vi "Get Sub Objects.vi"(8 "error in":errorcluster, 11 "Sub Objects Dictionary in":refnum<class "Sub Objects Dictionary.lvclass">) -> (0 "error out":errorcluster, 2 "Sub Objects":refnum<class "Sub Object.lvclass">[](array[class]), 3 "Sub Objects Dictionary out":refnum<class "Sub Objects Dictionary.lvclass">)   [LabVIEW 2020, in "CANopen.lvlib" / "Sub Objects Dictionary.lvclass"]
uses:
  Sub Objects Dictionary.lvclass
  Sub Objects Dictionary.lvclass/Sub Objects Dictionary.ctl
  Sub Object/Sub Object.lvclass
  Ordered-Dictionary/Ordered Object Dictionary/Source/Ordered Object Dictionary.lvclass
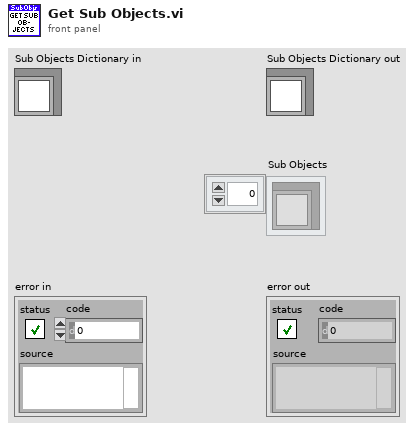
[diagram p1: front panel]
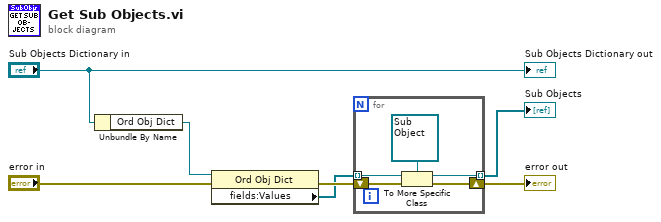
[diagram p0: block diagram]
diagram:
  n1 = Unbundle By Name("Sub Objects Dictionary in") -> ("Ord Obj Dict"=w4:refnum<class "Ordered Object Dictionary.lvclass">)
  n2 = property class="Ord Obj Dict"(reference=w4, error in="error in") -> (error out=w5:errorcluster, "fields:Values"=w1:refnum<class>[])  [unwired: 1 out]
  n3 = for {
    tunnel: w1 -> [w10] mode=indexing
    tunnel: [w9] -> w2 mode=indexing
    shift-right: [w11] -> w3
    shift-left: w5 -> [w12]
    n4 = To More Specific Class(target class=refnum<class "Sub Object.lvclass"> refnum ("CANopen.lvlib:Sub Obj"), reference=w10, error in=w12) -> (specific class reference=w9:refnum<class "Sub Object.lvclass">, error out=w11:errorcluster)
  }
  "error out" <- w3
  "Sub Objects" <- w2
  "Sub Objects Dictionary out" <- "Sub Objects Dictionary in"
